vi "TrendingWithHistogramm.vi"(0 "Data In":T4, 2 "Display State In":T2={"Sample Length"=0, "Index"=0, "Data Array"=[], "Intervals"=100, "Maximum"=0.0, "Minimum"=0.0, "Auto"=FALSE, "History Length"=1000}, 3 "Container State":T3) -> (6 "Data Out":T4, 7 "Display State Out":T2={"Sample Length"=0, "Index"=0, "Data Array"=[], "Intervals"=100, "Maximum"=0.0, "Minimum"=0.0, "Auto"=FALSE, "History Length"=1000}, 8 "Action":T1)   [LabVIEW 2014, in "TrendingWithHistogramm.xctl"]
doc: "1. Drop the controls that make up the appearance of the XControl here.\n2. Resize the window to fit the controls\n3. If the XControl is of fixed size, make the window not resizable from VI Properties->Window Appearance.\n4. If you want the controls to automatically size when the XControl sizes, check \"Scale all objects on front panel when window resizes\" in File->VI Properties->Window Size page.\n5. Show the block diagram and handle events for the controls on this panel."
uses:
  TrendingWithHistogramm.xctl
  Data.ctl
  <vilib>/_xctls/Container State.ctl
  State.ctl
  <vilib>/_xctls/Action.ctl
  <vilib>/_xctls/XControlSupport.lvlib
  <vilib>/ptbypt/NI_PtbyPt.lvlib
panel:
  in  "Clear":bool
  out "Long Term Trending":cluster{"mean":dbl, dbl, dbl, dbl, dbl}(graph)={"mean"=-0.10482093615145295, 0.8004682390195174, -1.0101101113224233, 2.2487016835526044, -2.2025195013609937}
  in  "Histogram Size":i32=600
  in  "Intervals":i32=10
  in  "Bind":bool
  out "Running Histogram":T5(graph)
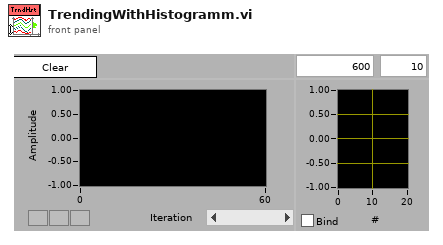
[diagram p1: front panel]
types:
  T1 = typedef "XControlSupport.lvlib/Action.ctl" = cluster{"Data Changed?":bool, "State Changed?":bool, "Action Name":string}
  T2 = typedef "TrendingWithHistogramm.xctl/State.ctl" = cluster{"Sample Length":i32, "Index":i32, "Data Array":dbl[], "Intervals":i32, "Maximum":dbl, "Minimum":dbl, "Auto":bool, "History Length":i32}
  T3 = typedef "XControlSupport.lvlib/Container State.ctl" = cluster{"Indicator?":bool, "Run Mode?":bool, " Refnum":refnum<vi>}
  T4 = typedef "TrendingWithHistogramm.xctl/Data.ctl" = dbl
  T5 = cluster{"Histogram: h(x)":i32[], "X Values":dbl[]}
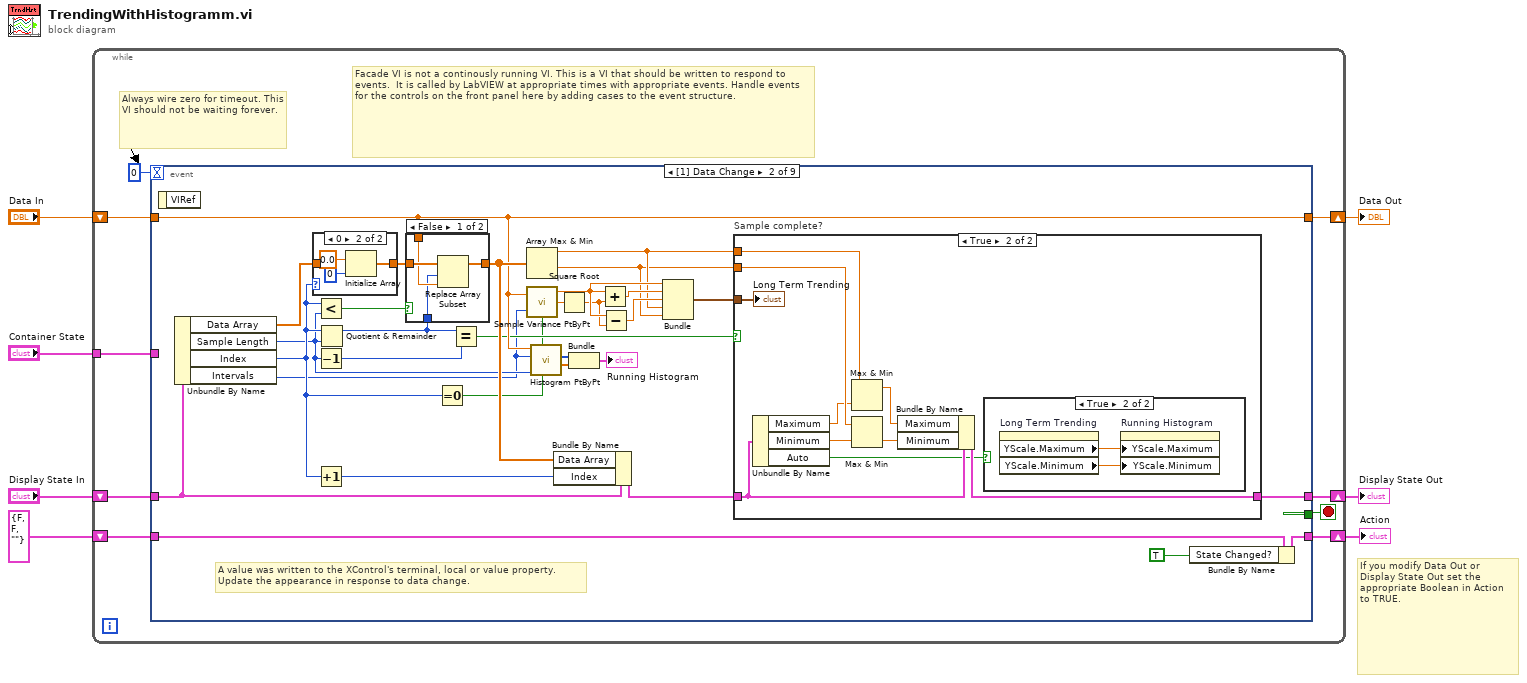
[diagram p0: block diagram]
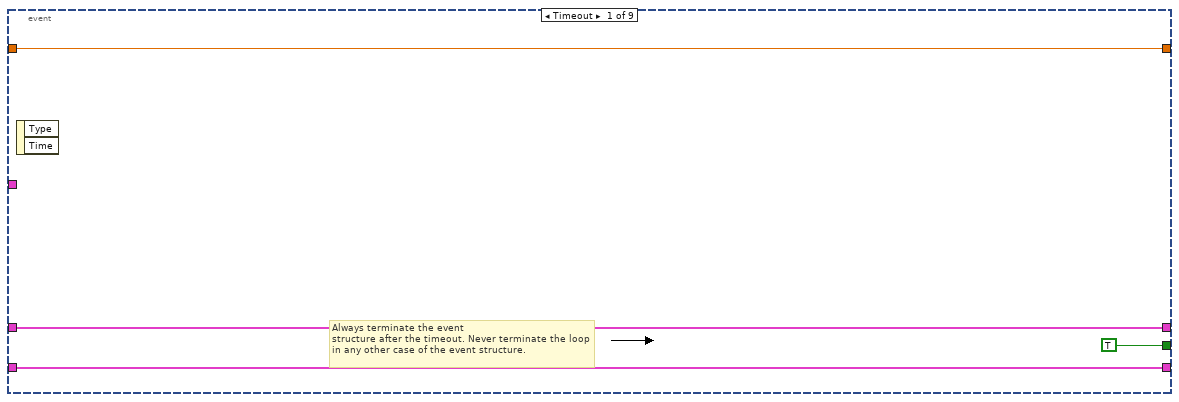
[diagram p2: hidden frame]
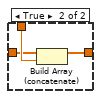
[diagram p5: hidden frame]
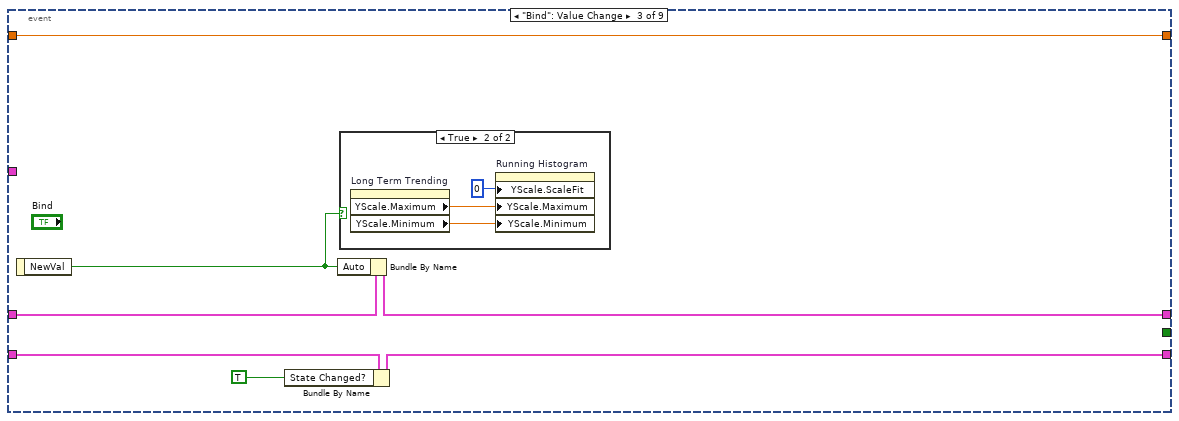
[diagram p7: hidden frame]
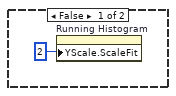
[diagram p8: hidden frame]
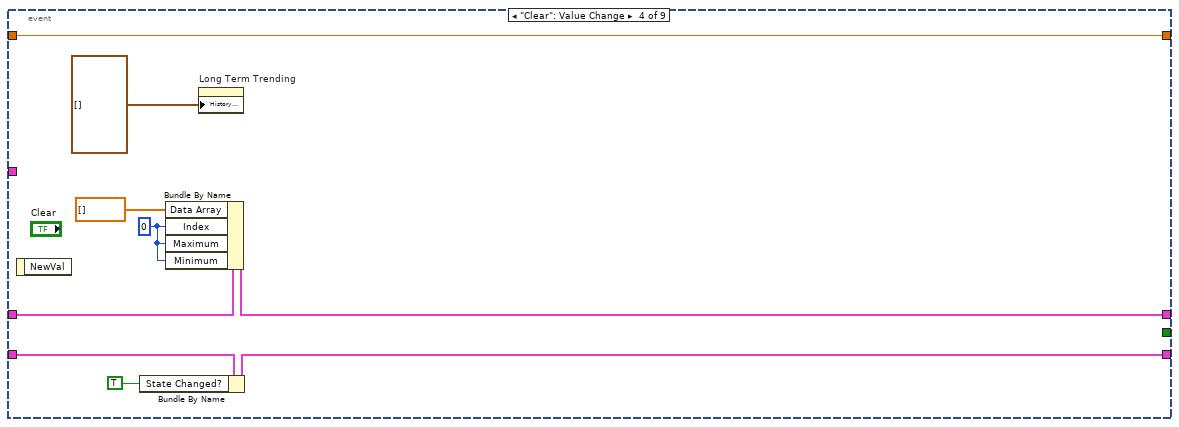
[diagram p9: hidden frame]
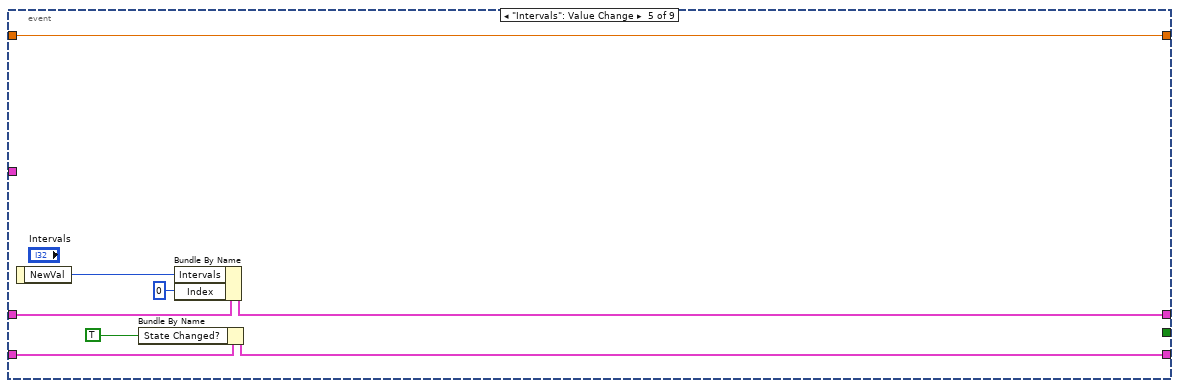
[diagram p10: hidden frame]
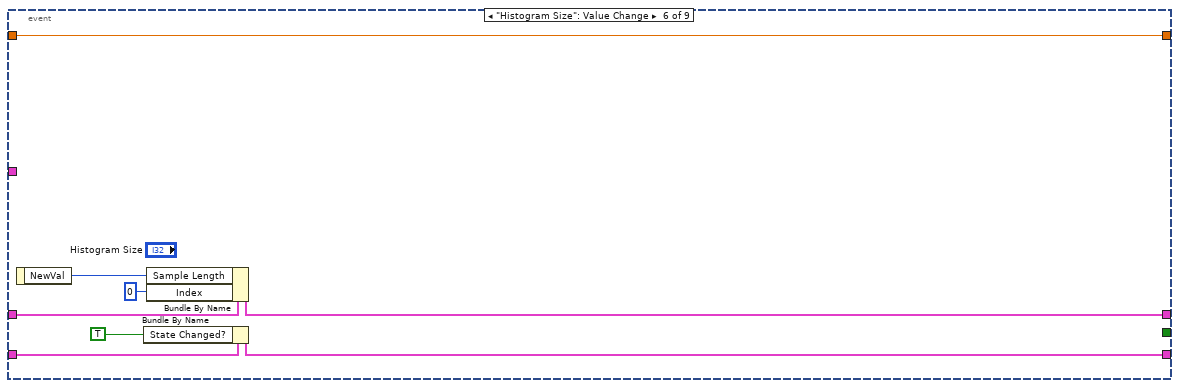
[diagram p11: hidden frame]
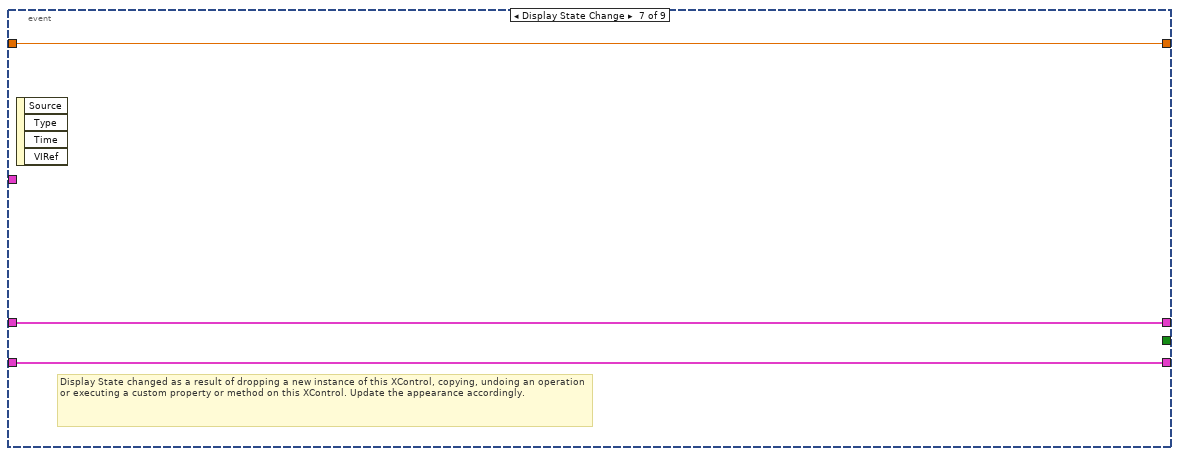
[diagram p12: hidden frame]
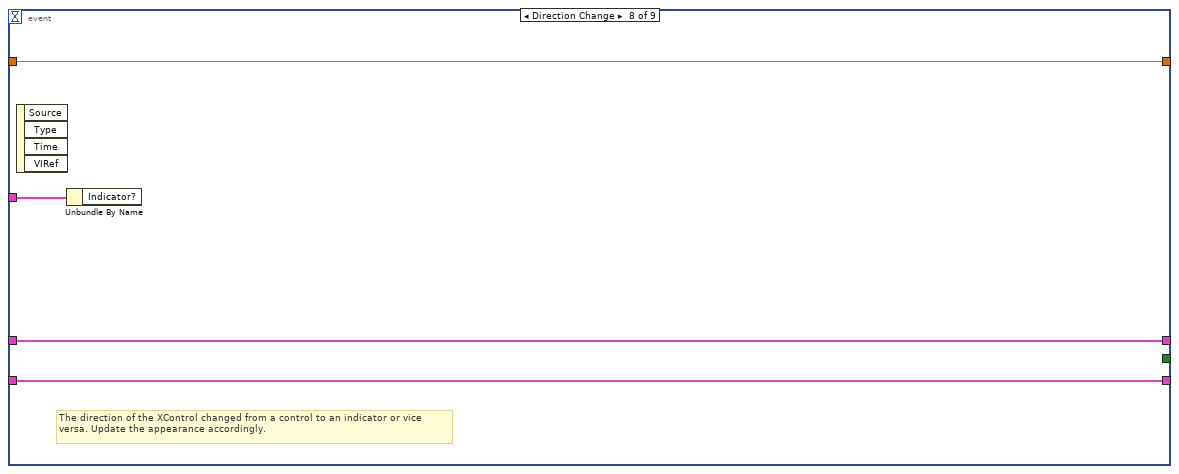
[diagram p13: hidden frame]
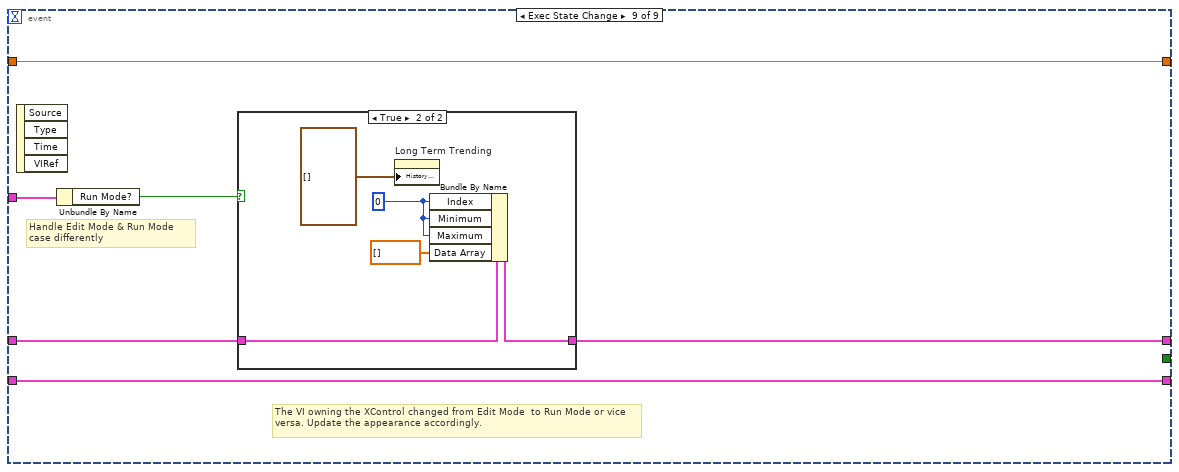
[diagram p14: hidden frame]
diagram:
  # "If you modify Data Out or\nDisplay State Out set the\nappropriate Boolean in Action\nto TRUE."
  n1 = while {
    shift-right: [w15] -> w4
    shift-left: "Display State In" -> [w16]
    tunnel: "Container State" -> [w12]
    shift-right: [w10] -> w7
    shift-left: "Data In" -> [w11]
    shift-right: [w8] -> w2
    shift-left: T1 {"Data Changed?"=FALSE, "State Changed?"=FALSE, "Action Name"=""} ("Action") -> [w9]
    stop <- w14 stop-if-true
    # "Facade VI is not a continously running VI. This is a VI that should be written to respond to events.  It is called by LabVIEW at appropriate times with appropriate events. Handle events for the controls on the front panel here by adding cases to the event structure."
    # "Always wire zero for timeout. This\nVI should not be waiting forever."
    n2 = event shown="[1] Data Change" {
      selector: _ -> [_ _ _ _ _ _ _ _ _]
      dyn-events: _ -> [_ _ _ _ _ _ _ _ _]
      timeout: 0 -> [_ _ _ _ _ _ _ _ _]
      tunnel: w16 -> [w18 w45 w77 w90 w102 w109 w113 w116 w120]
      tunnel: [w18 w24 w76 w89 w101 w108 w113 w116 w119] -> w15
      tunnel: [TRUE _ _ _ _ _ _ _ _] -> w14
      tunnel: w12 -> [_ _ _ _ _ _ _ w117 w123]
      tunnel: w11 -> [w17 w37 w81 w94 w99 w110 w112 w115 w122]
      tunnel: [w17 w37 w81 w94 w99 w110 w112 w115 w122] -> w10
      tunnel: [w19 w30 w78 w91 w96 w104 w111 w114 w121] -> w8
      tunnel: w9 -> [w19 w31 w79 w92 w97 w105 w111 w114 w121]
      event Timeout {
        # "Always terminate the event\nstructure after the timeout. Never terminate the loop in any other case of the event structure."
        n3 = event-data() -> ()  [unwired: 1 in, 2 out]
      }
      event Data Change {
        # "A value was written to the XControl's terminal, local or value property.\nUpdate the appearance in response to data change."
        n4 = event-data() -> ()  [unwired: 1 in, 1 out]
        n5 = Unbundle By Name(w45) -> ("Data Array"=w50:dbl[], "Sample Length"=w35:i32, "Index"=w36:i32, "Intervals"=w21:i32)
        n6 = case shown="0" w36 {
          tunnel: [w71 w73] -> w49
          tunnel: w50 -> [w71 _]
          frame Default {
          }
          frame 0 {
            n7 = Initialize Array(0.0 ("element"), 0 ("dimension size")) -> (w73:dbl[])
          }
        }
        n8 = Less?(x=w36, y=w35) -> (x < y?=w48:bool)
        n9 = Decrement(x=w35) -> (x-1=w47:i32)
        n10 = Increment(x=w36) -> (x+1=w44:i32)
        n11 = Quotient & Remainder(x=w36, y=w35) -> (x-y*floor(x/y)=w46:i32)  [unwired: 1 out]
        n12 = case shown="False" w48 {
          tunnel: w37 -> [w65 w70]
          tunnel: [w67 w69] -> w43
          tunnel: w49 -> [w66 w68]
          tunnel: w46 -> [w64 _]
          frame False {
            n13 = Replace Array Subset(array=w66, new element=w65, index=w64) -> (w67:dbl[])
          }
          frame True {
            n14 = Build Array (concatenate)(w68, w70) -> (w69:T4[])
          }
        }
        n15 = Equal To 0?(x=w36) -> (x = 0?=w22:bool)
        n16 = Equal?(x=w46, y=w47) -> (x = y?=w28:bool)
        n17 = Array Max & Min(array=w43) -> (max value=w27:T4, min value=w26:T4)  [unwired: 2 out]
        n18 = call <vilib>:"Sample Variance PtByPt.vi"("x"=w37, "sample length"=w21, "initialize"=w22) -> ("mean"=w40:dbl, "sample variance"=w41:dbl)  [unwired: 1 out]
        n19 = call <vilib>:"Histogram PtByPt.vi"("initialize"=w22, "sample length"=w35, "intervals"=w21, "x"=w37) -> ("X Values"=w38:dbl[], "Histogram: h(x)"=w34:i32[])  [unwired: 4 in, 2 out]
        n20 = Bundle By Name(cluster=w45, "Data Array"=w43, "Index"=w44) -> (w25:T2)
        n21 = Square Root(x=w41) -> (sqrt(x)=w23:dbl)
        n22 = Bundle("Histogram: h(x)"=w34, "X Values"=w38) -> (→"Running Histogram":T5)  [unwired: 1 in]
        n23 = Add(x=w40, y=w23) -> (x+y=w39:dbl)
        n24 = Subtract(x=w40, y=w23) -> (x-y=w42:dbl)
        n25 = Bundle("mean"=w40, w39, w42, w27, w26) -> (w32:cluster{"mean":dbl, dbl, dbl, T4, T4})  [unwired: 1 in]
        n26 = case "Sample complete?" shown="True" w28 {
          tunnel: w32 -> [_ w61]
          tunnel: w27 -> [_ w60]
          tunnel: w26 -> [_ w57]
          tunnel: w25 -> [w51 w59]
          tunnel: [w51 w58] -> w24
          frame False {
          }
          frame True {
            n27 = Unbundle By Name(w59) -> ("Maximum"=w54:dbl, "Minimum"=w56:dbl, "Auto"=w52:bool)
            n28 = Max & Min(x=w60, y=w54) -> (max(x,y)=w53:T4)  [unwired: 1 out]
            n29 = Max & Min(x=w57, y=w56) -> (min(x,y)=w55:T4)  [unwired: 1 out]
            n30 = Bundle By Name(cluster=w59, "Maximum"=w53, "Minimum"=w55) -> (w58:T2)
            n31 = case shown="True" w52 {
              frame False {
              }
              frame True {
                n32 = property on="Long Term Trending" class="WFChart (strict)"() -> ("YScale.Maximum"=w63:dbl, "YScale.Minimum"=w62:dbl)  [unwired: 2 in, 2 out]
                n33 = property on="Running Histogram" class="XYGraph (strict)"("YScale.Maximum"=w63, "YScale.Minimum"=w62) -> ()  [unwired: 2 in, 2 out]
              }
            }
            "Long Term Trending" <- w61
          }
        }
        n34 = Bundle By Name(cluster=w31, "State Changed?"=TRUE) -> (w30:T1)
      }
      event "Bind": Value Change {
        n35 = event-data() -> ("NewVal"=w75:bool)  [unwired: 1 in]
        n36 = Bundle By Name(cluster=w79, "State Changed?"=TRUE) -> (w78:T1)
        n37 = Bundle By Name(cluster=w77, "Auto"=w75) -> (w76:T2)
        n38 = case shown="True" w75 {
          frame False {
            n39 = property on="Running Histogram" class="XYGraph (strict)"("YScale.ScaleFit"=u8 2 ("Y Scale.Scale Fit")) -> ()  [unwired: 2 in, 2 out]
          }
          frame True {
            n40 = property on="Long Term Trending" class="WFChart (strict)"() -> ("YScale.Maximum"=w85:dbl, "YScale.Minimum"=w84:dbl)  [unwired: 2 in, 2 out]
            n41 = property on="Running Histogram" class="XYGraph (strict)"("YScale.ScaleFit"=u8 0 ("Y Scale.Scale Fit"), "YScale.Maximum"=w85, "YScale.Minimum"=w84) -> ()  [unwired: 2 in, 2 out]
          }
        }
      }
      event "Clear": Value Change {
        w87 = 0 ("Index")
        n42 = event-data() -> ()  [unwired: 1 in, 1 out]
        n43 = Bundle By Name(cluster=w92, "State Changed?"=TRUE) -> (w91:T1)
        n44 = Bundle By Name(cluster=w90, "Data Array"=dbl[] [], "Index"=w87, "Maximum"=w87, "Minimum"=w87) -> (w89:T2)
        n45 = property on="Long Term Trending" class="WFChart (strict)"("History Data"=cluster{"mean":dbl, dbl, dbl, dbl, dbl}[] []) -> ()  [unwired: 2 in, 2 out]
      }
      event "Intervals": Value Change {
        n46 = event-data() -> ("NewVal"=w100:i32)  [unwired: 1 in]
        n47 = Bundle By Name(cluster=w97, "State Changed?"=TRUE) -> (w96:T1)
        n48 = Bundle By Name(cluster=w102, "Intervals"=w100, "Index"=0) -> (w101:T2)
      }
      event "Histogram Size": Value Change {
        n49 = event-data() -> ("NewVal"=w107:i32)  [unwired: 1 in]
        n50 = Bundle By Name(cluster=w105, "State Changed?"=TRUE) -> (w104:T1)
        n51 = Bundle By Name(cluster=w109, "Sample Length"=w107, "Index"=0) -> (w108:T2)
      }
      event Display State Change {
        # "Display State changed as a result of dropping a new instance of this XControl, copying, undoing an operation or executing a custom property or method on this XControl. Update the appearance accordingly."
        n52 = event-data() -> ()  [unwired: 1 in, 4 out]
      }
      event Direction Change {
        # "The direction of the XControl changed from a control to an indicator or vice versa. Update the appearance accordingly."
        n53 = event-data() -> ()  [unwired: 1 in, 4 out]
        n54 = Unbundle By Name(w117) -> ()  [unwired: 1 out]
      }
      event Exec State Change {
        # "The VI owning the XControl changed from Edit Mode  to Run Mode or vice versa. Update the appearance accordingly."
        # "Handle Edit Mode & Run Mode\ncase differently"
        n55 = event-data() -> ()  [unwired: 1 in, 4 out]
        n56 = Unbundle By Name(w123) -> ("Run Mode?"=w118:bool)
        n57 = case shown="True" w118 {
          tunnel: w120 -> [w124 w129]
          tunnel: [w124 w128] -> w119
          frame False {
          }
          frame True {
            w126 = 0 ("Index")
            n58 = property on="Long Term Trending" class="WFChart (strict)"("History Data"=cluster{"mean":dbl, dbl, dbl, dbl, dbl}[] []) -> ()  [unwired: 2 in, 2 out]
            n59 = Bundle By Name(cluster=w129, "Index"=w126, "Minimum"=w126, "Maximum"=w126, "Data Array"=dbl[] []) -> (w128:T2)
          }
        }
      }
    }
  }
  "Display State Out" <- w4
  "Data Out" <- w7
  "Action" <- w2
